vi "Set_Hardware.vi"(8 "error in (no error)":errorcluster, 11 "Control in":refnum<class "Control-Server.lvclass">) -> (0 "error out":errorcluster, 3 "Control out":refnum<class "Control-Server.lvclass">)   [LabVIEW 2015, in "Control-Server.lvclass"]
uses:
  Control-Server.lvclass
  dependecies/ControlsVIs/Clusters-def/Message types.ctl
  Message/Message.lvclass
  Message/Message.lvclass/Message.ctl
  GeneralFunctionality/GeneralFunctionality.lvclass
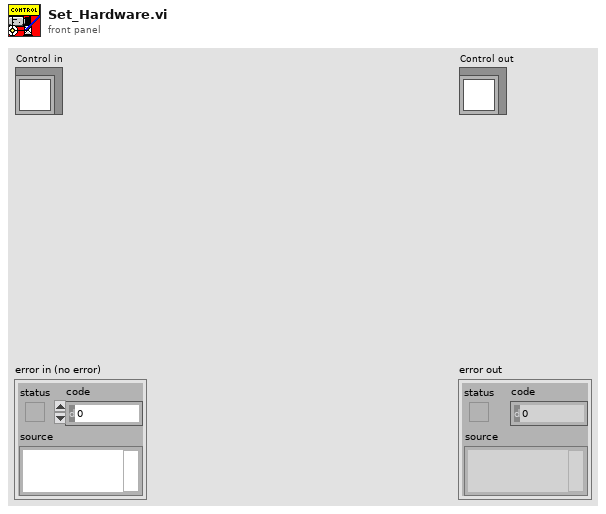
[diagram p1: front panel]
types:
  T1 = typedef "Message types.ctl" = string
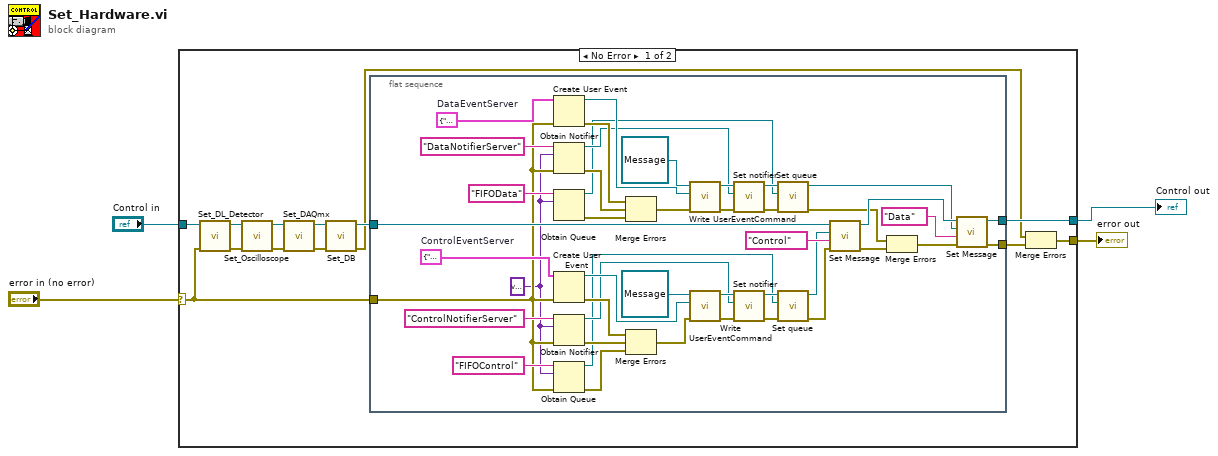
[diagram p0: block diagram]
diagram:
  n1 = case shown="No Error" "error in (no error)" {
    selector: "error in (no error)" -> [w15 w62]
    tunnel: [w13 w62] -> w3
    tunnel: [w16 w63] -> w1
    tunnel: "Control in" -> [w17 w63]
    frame No Error {
      n2 = call "Set_DL_Detector.vi"("error in (no error)"=w15, "Control-Server in"=w17) -> ("error out"=w12:errorcluster, "Control-Server out"=w11:refnum<class "Control-Server.lvclass">)  [unwired: 8 in]
      n3 = call "Set_Oscilloscope.vi"("error in (no error)"=w12, "Control-Server in"=w11) -> ("error out"=w9:errorcluster, "Control-Server out"=w10:refnum<class "Control-Server.lvclass">)  [unwired: 8 in]
      n4 = call "Set_DAQmx.vi"("error in (no error)"=w9, "Control-Server in"=w10) -> ("error out"=w5:errorcluster, "Control-Server out"=w8:refnum<class "Control-Server.lvclass">)  [unwired: 8 in]
      n5 = call "Set_DB.vi"("error in (no error)"=w5, "Control-Server in"=w8) -> ("error out"=w6:errorcluster, "Control-Server out"=w7:refnum<class "Control-Server.lvclass">)  [unwired: 8 in]
      n6 = flat-sequence {
        tunnel: w7 -> [w51]
        tunnel: [w20] -> w16
        tunnel: [w21] -> w14
        tunnel: w15 -> [w19]
        frame #0 {
          w39 = cluster{"command":string, "data":variant} {"command"="", "data"=variant}  # DataEventServer
          w18 = variant
          w57 = cluster{"command":string, "data":variant} {"command"="", "data"=variant}  # ControlEventServer
          n7 = Create User Event(user event datatype=w39, error in=w19) -> (user event=w32:refnum<user-event>, error out=w37:errorcluster)
          n8 = Obtain Notifier(name (unnamed)="DataNotifierServer" ("nom (aucun)"), notification data type=w18, error in (no error)=w19) -> (notifier out=w31:refnum<notifier>, error out=w36:errorcluster)  [unwired: 1 in, 1 out]
          n9 = Obtain Queue(name (unnamed)="FIFOData", element data type=w18) -> (queue out=w28:refnum<queue>, error out=w34:errorcluster)  [unwired: 3 in, 1 out]
          n10 = Create User Event(user event datatype=w57, error in=w19) -> (user event=w59:refnum<user-event>, error out=w55:errorcluster)
          n11 = Obtain Notifier(name (unnamed)="ControlNotifierServer" ("nom (aucun)"), notification data type=w18, error in (no error)=w19) -> (notifier out=w53:refnum<notifier>, error out=w54:errorcluster)  [unwired: 1 in, 1 out]
          n12 = Obtain Queue(name (unnamed)="FIFOControl", element data type=w18, error in (no error)=w19) -> (queue out=w29:refnum<queue>, error out=w35:errorcluster)  [unwired: 2 in, 1 out]
          n13 = Merge Errors(w37, w36, w34) -> (w33:errorcluster)
          n14 = Merge Errors(w55, w54, w35) -> (w52:errorcluster)
          n15 = call "Write UserEventCommand.vi"("error in (no error)"=w33, "UserEventCommand"=w32, "Message en entrée"=refnum<class "Message.lvclass"> refnum ("Message.lvclass")) -> ("error out"=w43:errorcluster, "Message en sortie"=w42:refnum<class "Message.lvclass">)  [unwired: 7 in]
          n16 = call "Write UserEventCommand.vi"("error in (no error)"=w52, "UserEventCommand"=w59, "Message en entrée"=refnum<class "Message.lvclass"> refnum ("Message.lvclass")) -> ("error out"=w56:errorcluster, "Message en sortie"=w60:refnum<class "Message.lvclass">)  [unwired: 7 in]
          n17 = call "Set notifier.vi"("error in (no error)"=w43, "notifier"=w31, "Message en entrée"=w42) -> ("error out"=w30:errorcluster, "Message en sortie"=w40:refnum<class "Message.lvclass">)  [unwired: 7 in]
          n18 = call "Set notifier.vi"("error in (no error)"=w56, "notifier"=w53, "Message en entrée"=w60) -> ("error out"=w48:errorcluster, "Message en sortie"=w49:refnum<class "Message.lvclass">)  [unwired: 7 in]
          n19 = call "Set queue.vi"("error in (no error)"=w30, "queue"=w28, "Message in"=w40) -> ("error out"=w25:errorcluster, "Message out"=w26:refnum<class "Message.lvclass">)  [unwired: 7 in]
          n20 = call "Set queue.vi"("error in (no error)"=w48, "queue"=w29, "Message in"=w49) -> ("error out"=w46:errorcluster, "Message out"=w45:refnum<class "Message.lvclass">)  [unwired: 7 in]
          n21 = call "Set Message.vi"("error in (no error)"=w46, "Message type"=T1 "Control", "Message.lvclass"=w45, "GeneralFunctionality en entrée"=w51) -> ("error out"=w24:errorcluster, "GeneralFunctionality en sortie"=w27:refnum<class "Control-Server.lvclass">)  [unwired: 6 in]
          n22 = Merge Errors(w25, w24) -> (w23:errorcluster)
          n23 = call "Set Message.vi"("error in (no error)"=w23, "Message type"=T1 "Data", "Message.lvclass"=w26, "GeneralFunctionality en entrée"=w27) -> ("error out"=w21:errorcluster, "GeneralFunctionality en sortie"=w20:refnum<class "Control-Server.lvclass">)  [unwired: 6 in]
        }
      }
      n24 = Merge Errors(w6, w14) -> (w13:errorcluster)
    }
    frame Error {
    }
  }
  "error out" <- w3
  "Control out" <- w1
